vi "getParAndArgChkRes_.vi"(8 "error in":errorcluster, 9 "func":string, 10 "arg":string, 11 "Tree Refnum in":refnum<vi>) -> (0 "error out":errorcluster, 1 "Check result":string="√", 2 "par":string, 3 "Tree Refnum out":refnum<vi>)   [LabVIEW 2010]
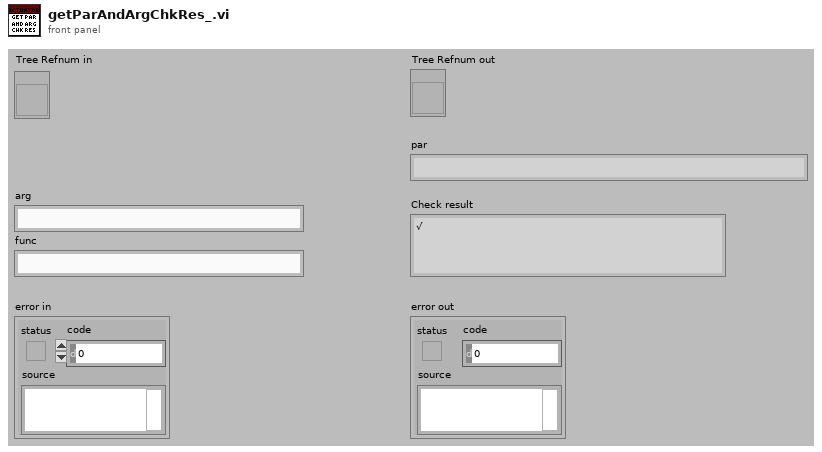
[diagram p1: front panel]
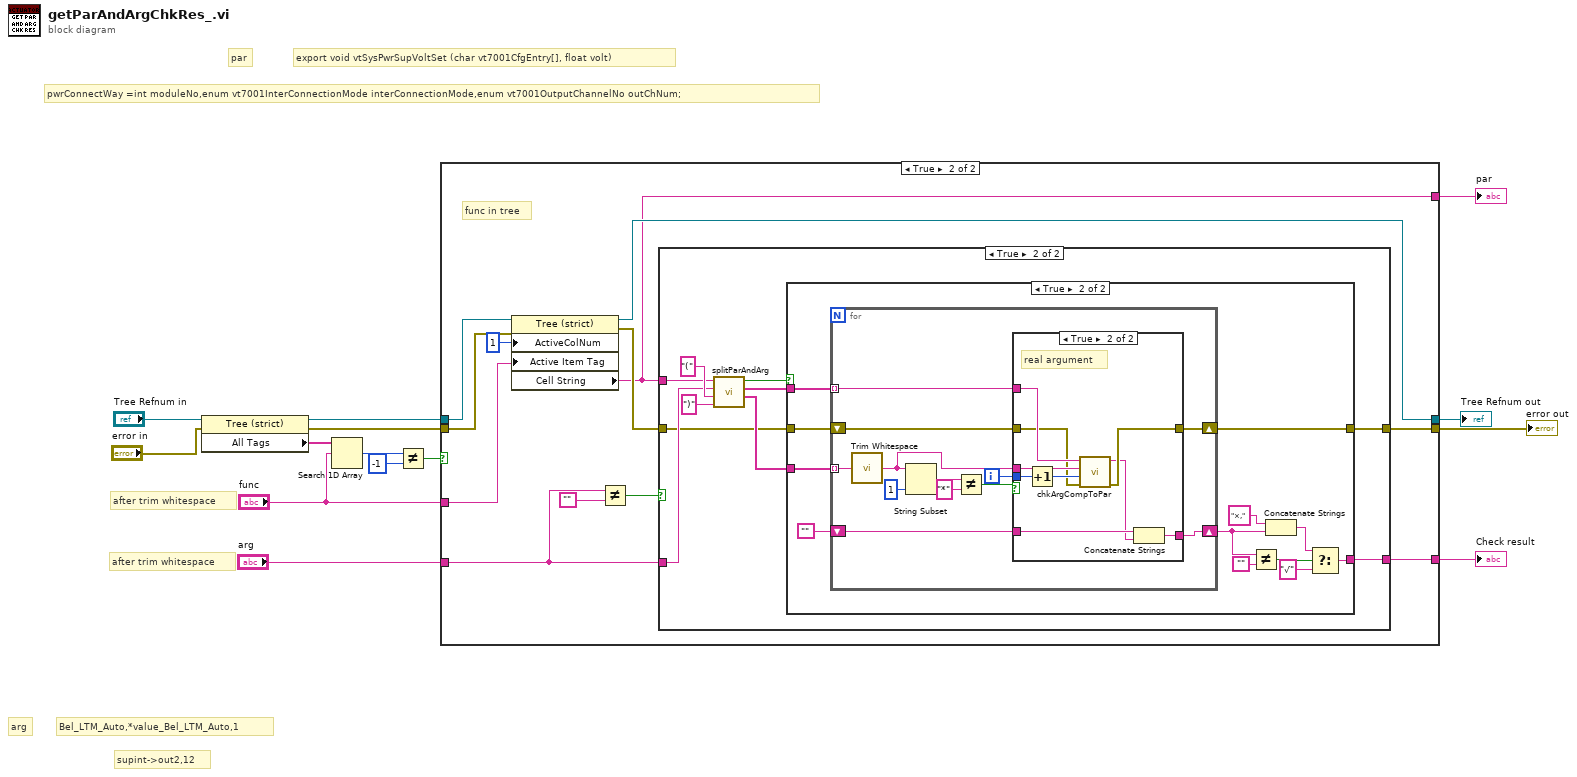
[diagram p0: block diagram]
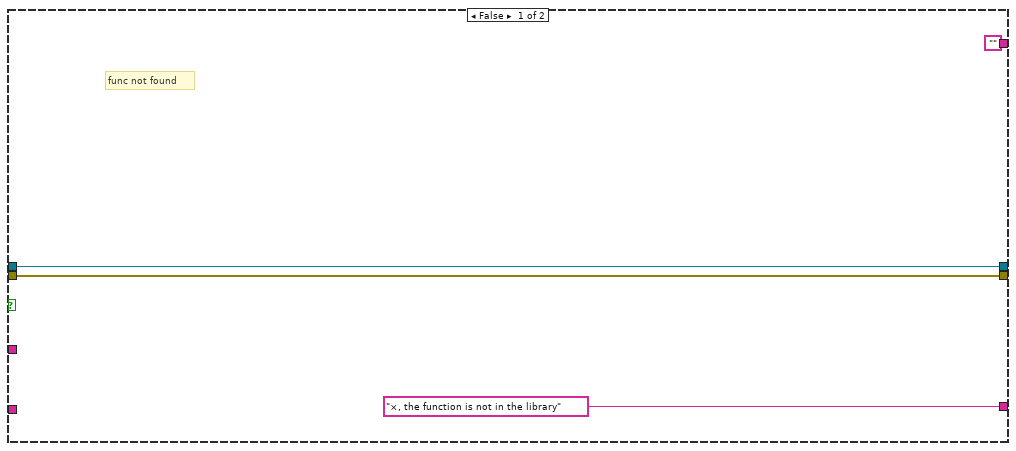
[diagram p2: hidden frame]
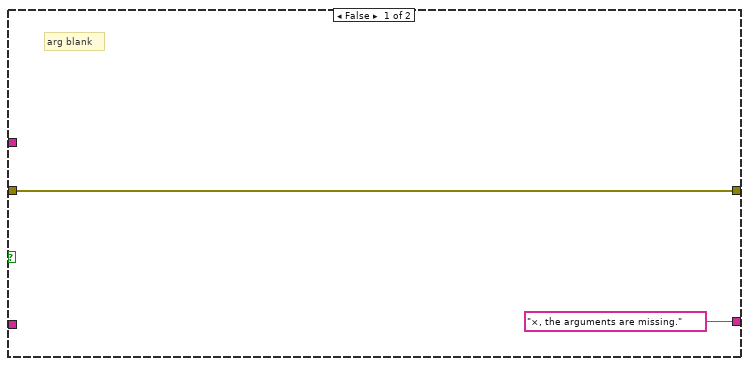
[diagram p3: hidden frame]
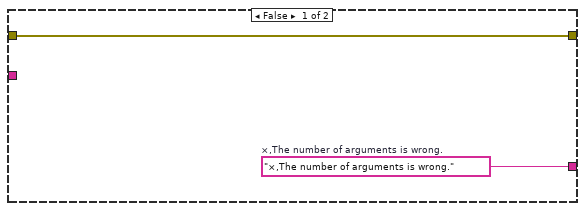
[diagram p4: hidden frame]
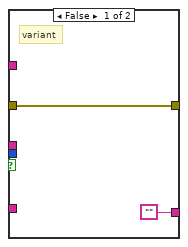
[diagram p5: hidden frame]
diagram:
  # "after trim whitespace"
  # "after trim whitespace"
  # "pwrConnectWay =int moduleNo,enum vt7001InterConnectionMode interConnectionMode,enum vt7001OutputChannelNo outChNum;"
  # "arg"
  # "par"
  # "Bel_LTM_Auto,*value_Bel_LTM_Auto,1"
  # "supint->out2,12"
  # "export void vtSysPwrSupVoltSet (char vt7001CfgEntry[], float volt)"
  n1 = property on="Property Node" class="Tree (strict)"(reference="Tree Refnum in", error in="error in") -> (reference out=w7:refnum<vi>, error out=w8:errorcluster, "All Tags"=w11:string[])
  n2 = Search 1D Array(1D array=w11, element="func") -> (index of element=w10:i32)  [unwired: 1 in]
  n3 = Not Equal?(x=w10, y=-1) -> (x != y?=w14:bool)
  n4 = case shown="True" w14 {
    tunnel: "arg" -> [_ w19]
    tunnel: w8 -> [w16 w25]
    tunnel: ["×, the function is not in the library" w30] -> w13
    tunnel: [w16 w29] -> w12
    tunnel: w7 -> [w17 w23]
    tunnel: [w17 w21] -> w6
    tunnel: "func" -> [_ w24]
    tunnel: ["" w20] -> w3
    frame False {
      # "func not found"
    }
    frame True {
      # "func in tree"
      n5 = property class="Tree (strict)"(reference=w23, error in=w25, "ActiveColNum"=1 ("Active Cell:Active Column Number"), "Active Item Tag"=w24) -> (reference out=w21:refnum<vi>, error out=w22:errorcluster, "Cell String"=w20:string)
      n6 = Not Equal?(x=w19, y="") -> (x != y?=w27:bool)
      n7 = case shown="True" w27 {
        tunnel: w20 -> [_ w38]
        tunnel: w19 -> [_ w37]
        tunnel: w22 -> [w32 w33]
        tunnel: ["×, the arguments are missing." w42] -> w30
        tunnel: [w32 w41] -> w29
        frame False {
          # "arg blank"
        }
        frame True {
          n8 = call "splitParAndArg.vi"("paraEndMark"=")" ("regular expression"), "paraStartMark"="(" ("regular expression"), "allArguments"=w37, "allParameters"=w38) -> ("argArray"=w35:string[], "paraArray"=w36:string[], "sameNum?"=w34:bool)  [unwired: 5 in]
          n9 = case shown="True" w34 {
            tunnel: w36 -> [_ w56]
            tunnel: w35 -> [_ w55]
            tunnel: [w44 w50] -> w42
            tunnel: w33 -> [w43 w49]
            tunnel: [w43 w48] -> w41
            frame False {
              w44 = "×,The number of arguments is wrong."  # ×,The number of arguments is wrong.
            }
            frame True {
              n10 = for {
                tunnel: w56 -> [w68] mode=indexing
                tunnel: w55 -> [w58] mode=indexing
                shift-right: [w66] -> w46
                shift-left: "" -> [w67]
                shift-right: [w64] -> w48
                shift-left: w49 -> [w65]
                i -> [w59]
                n11 = call <vilib>:"Trim Whitespace.vi"("string"=w58) -> ("trimmed string"=w57:string)  [unwired: 1 in]
                n12 = String Subset(string=w57, length (rest)=1 ("length (rest)")) -> (substring=w62:string)  [unwired: 1 in]
                n13 = Not Equal?(x=w62, y="*") -> (x != y?=w60:bool)
                n14 = case shown="True" w60 {
                  tunnel: w68 -> [_ w76]
                  tunnel: w67 -> [_ w79]
                  tunnel: ["" w78] -> w66
                  tunnel: w65 -> [w69 w73]
                  tunnel: [w69 w72] -> w64
                  tunnel: w59 -> [_ w75]
                  tunnel: w57 -> [_ w77]
                  frame False {
                    # "variant"
                  }
                  frame True {
                    # "real argument"
                    n15 = Increment(x=w75) -> (x+1=w74:i32)
                    n16 = call "chkArgCompToPar.vi"("error in"=w73, "argSN"=w74, "arg"=w77, "par"=w76) -> ("error out"=w72:errorcluster, "judgement"=w71:string)  [unwired: 6 in]
                    n17 = Concatenate Strings(w79, w71) -> (w78:string)
                  }
                }
              }
              n18 = Not Equal?(x=w46, y="") -> (x != y?=w52:bool)
              n19 = Concatenate Strings("×,", w46) -> (w45:string)
              n20 = Select(t=w45, s=w52, f="√") -> (s? t:f=w50:string)
            }
          }
        }
      }
    }
  }
  "Check result" <- w13
  "error out" <- w12
  "Tree Refnum out" <- w6
  "par" <- w3
